vi "message generator.vi"(8 "error in":errorcluster, 10 "data":string="Welcome Message", 11 "message":string="Welcome Message") -> (0 "error out":errorcluster, 1 "Message":string, 2 "Right Menu":T1, 3 "Left Menu":T1)   [LabVIEW 2015]
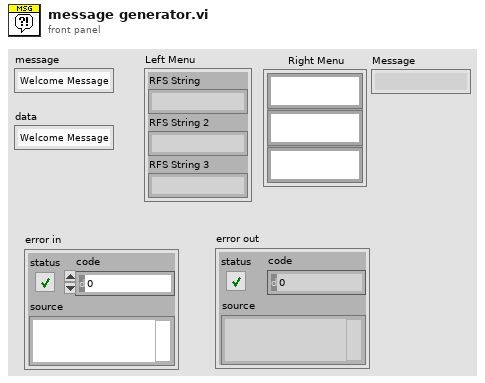
[diagram p1: front panel]
types:
  T1 = cluster{"RFS String":string, "RFS String 2":string, "RFS String 3":string}
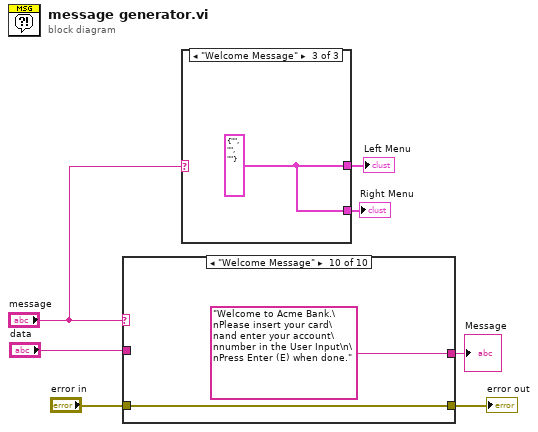
[diagram p0: block diagram]
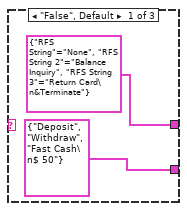
[diagram p2: hidden frame]
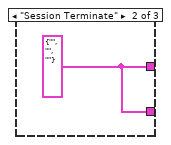
[diagram p3: hidden frame]
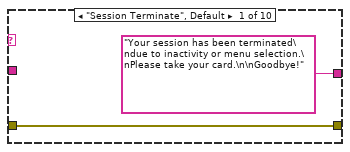
[diagram p4: hidden frame]
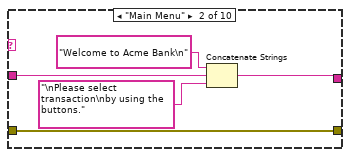
[diagram p5: hidden frame]
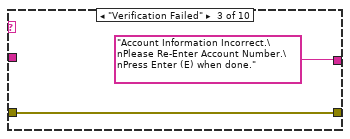
[diagram p6: hidden frame]
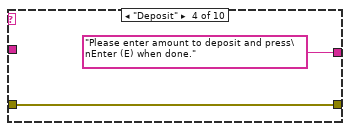
[diagram p7: hidden frame]
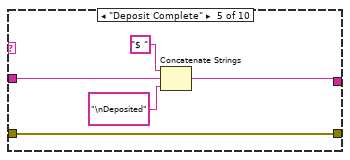
[diagram p8: hidden frame]
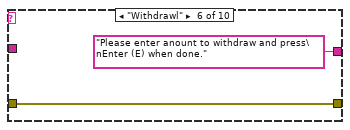
[diagram p9: hidden frame]
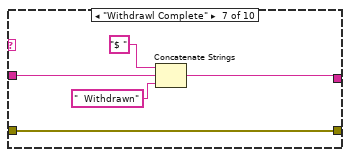
[diagram p10: hidden frame]
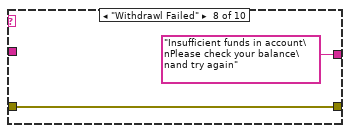
[diagram p11: hidden frame]
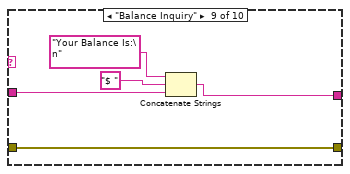
[diagram p12: hidden frame]
diagram:
  n1 = case shown="\"Welcome Message\"" "message" {
    tunnel: ["Your session has been terminated\ndue to inactivity or menu selection.\nPlease take your card.\n\nGoodbye!" w11 "Account Information Incorrect.\nPlease Re-Enter Account Number.\nPress Enter (E) when done." "Please enter amount to deposit and press\nEnter (E) when done." w20 "Please enter anount to withdraw and press\nEnter (E) when done." w27 "Insufficient funds in account\nPlease check your balance\nand try again" w34 "Welcome to Acme Bank.\nPlease insert your card\nand enter your account\nnumber in the User Input\n\nPress Enter (E) when done."] -> w4
    tunnel: "data" -> [_ w13 _ _ w21 _ w29 _ w35 _]
    tunnel: [w8 w10 w15 w17 w19 w24 w26 w31 w33 w38] -> w2
    tunnel: "error in" -> [w8 w10 w15 w17 w19 w24 w26 w31 w33 w38]
    frame "Session Terminate", Default {
    }
    frame "Main Menu" {
      n2 = Concatenate Strings("Welcome to Acme Bank\n", w13, "\nPlease select transaction\nby using the buttons.") -> (w11:string)
    }
    frame "Verification Failed" {
    }
    frame "Deposit" {
    }
    frame "Deposit Complete" {
      n3 = Concatenate Strings("$ " ("string"), w21, "\nDeposited" ("string")) -> (w20:string)
    }
    frame "Withdrawl" {
    }
    frame "Withdrawl Complete" {
      n4 = Concatenate Strings("$ ", w29, "  Withdrawn" ("string")) -> (w27:string)
    }
    frame "Withdrawl Failed" {
    }
    frame "Balance Inquiry" {
      n5 = Concatenate Strings("Your Balance Is:\n" ("string"), "$ " ("string"), w35) -> (w34:string)
    }
    frame "Welcome Message" {
    }
  }
  "Message" <- w4
  "error out" <- w2
  n6 = case shown="\"Welcome Message\"" "message" {
    tunnel: [T1 {"RFS String"="None", "RFS String 2"="Balance Inquiry", "RFS String 3"="Return Card\n&Terminate"} ("Left Menu") w42 w43] -> w6
    tunnel: [T1 {"RFS String"="Deposit", "RFS String 2"="Withdraw", "RFS String 3"="Fast Cash\n$ 50"} ("Left Menu") w42 w43] -> w7
    frame "False", Default {
    }
    frame "Session Terminate" {
      w42 = T1 {"RFS String"="", "RFS String 2"="", "RFS String 3"=""} ("Left Menu")
    }
    frame "Welcome Message" {
      w43 = T1 {"RFS String"="", "RFS String 2"="", "RFS String 3"=""} ("Left Menu")
    }
  }
  "Left Menu" <- w6
  "Right Menu" <- w7
